vi "tcp_client.vi"() -> ()   [LabVIEW 2013]
panel:
  in  "Disconnect From Server":bool
  in  "Read From Server":bool
  in  "IP address":string
  out "Recevied Value":T1 {"Word 3" format="%x"; "Word 2" format="%x"; "Word 1" format="%x"}
  out "error out":errorcluster
  in  "Port":u16
  # "Basic client server test.  Labview is the client. Run to connect, then use the two buttons below to read\nfrom the server and/or disconnect.  The server is set up now to just send sequential numbers - this \nis a placeholder until it actually does some processing."
  # "IP Address might be 127.0.0.1 to test a server running on the same machine as Labview\nOr it could be the IP address of the TK1 board once that is up and running"
  # "Port is arbitrary - make it a number above 49152. Start the server using that same port number. It has to be unique on the machine running the server, but not unique over the whole internet."
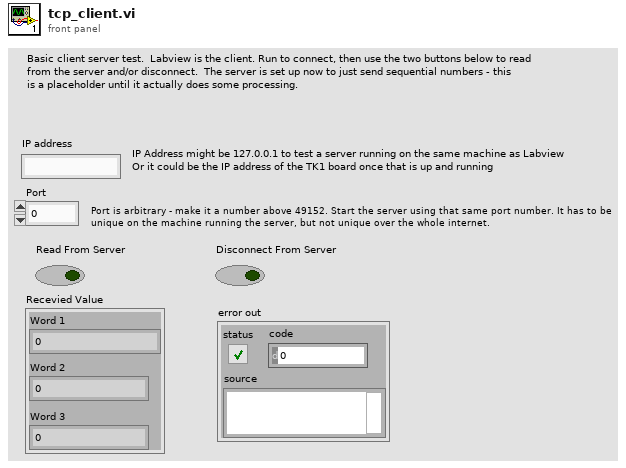
[diagram p1: front panel]
types:
  T1 = cluster{"Word 1":u32, "Word 2":u32, "Word 3":u32}
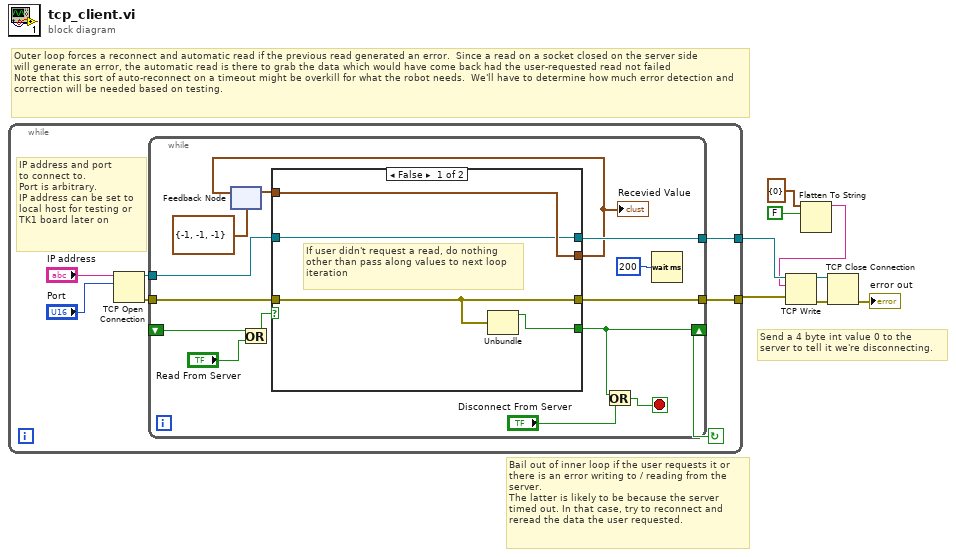
[diagram p0: block diagram]
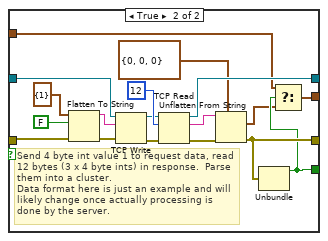
[diagram p2: hidden frame]
diagram:
  # "Send a 4 byte int value 0 to the\nserver to tell it we're disconnecting."
  # "Bail out of inner loop if the user requests it or\nthere is an error writing to / reading from the \nserver.\nThe latter is likely to be because the server\ntimed out. In that case, try to reconnect and \nreread the data the user requested."
  # "Outer loop forces a reconnect and automatic read if the previous read generated an error.  Since a read on a socket closed on the server side\nwill generate an error, the automatic read is there to grab the data which would have come back had the user-requested read not failed\nNote that this sort of auto-reconnect on a timeout might be overkill for what the robot needs.  We'll have to determine how much error detection and correction will be needed based on testing."
  n1 = while {
    tunnel: [w11] -> w3
    tunnel: [w10] -> w2
    stop <- w9 continue-if-true
    # "IP address and port\nto connect to.\nPort is arbitrary.\nIP address can be set to local host for testing or\nTK1 board later on"
    n2 = TCP Open Connection(address="IP address", remote port or service name="Port") -> (connection ID=w12:refnum<k5>, error out=w13:errorcluster)  [unwired: 3 in]
    n3 = while {
      tunnel: w13 -> [w29]
      tunnel: w12 -> [w28]
      tunnel: [w25] -> w11
      tunnel: [w26] -> w10
      shift-right: [w18] -> w9
      shift-left: _ -> [w21]
      stop <- w24 stop-if-true
      n4 = feedback #1(cluster{i32, i32, i32} {-1, -1, -1}) -> (w19:cluster{u32, u32, u32})
      n5 = Or(x=w21, y="Read From Server") -> (x .or. y?=w20:bool)
      n6 = case shown="False" w20 {
        tunnel: [w33 w36] -> w17
        tunnel: w29 -> [w31 w40]
        tunnel: w28 -> [w32 w49]
        tunnel: [w32 w46] -> w26
        tunnel: [w31 w38] -> w25
        tunnel: w19 -> [w33 w35]
        tunnel: [w30 w37] -> w18
        frame False {
          # "If user didn't request a read, do nothing\nother than pass along values to next loop\niteration"
          n7 = Unbundle(w31) -> ("status"=w30:bool)  [unwired: 2 out]
        }
        frame True {
          # "Send 4 byte int value 1 to request data, read 12 bytes (3 x 4 byte ints) in response.  Parse them into a cluster.  \nData format here is just an example and will likely change once actually processing is done by the server."
          n8 = Flatten To String(anything=cluster{u32} {1}, prepend array or string size? (T)=FALSE, error in (no error)=w40) -> (data string=w43:string, error out=w39:errorcluster)  [unwired: 1 in, 1 out]
          n9 = TCP Write(connection ID=w49, data in=w43, error in (no error)=w39) -> (connection ID out=w48:refnum<k5>, error out=w47:errorcluster)  [unwired: 1 in, 1 out]
          n10 = TCP Read(connection ID=w48, bytes to read=12, error in (no error)=w47) -> (connection ID out=w46:refnum<k5>, data out=w50:string, error out=w41:errorcluster)  [unwired: 2 in]
          n11 = Unflatten From String(type=cluster{u32, u32, u32} {0, 0, 0}, binary string=w50, error in (no error)=w41) -> (value=w34:cluster{u32, u32, u32}, error out=w38:errorcluster)  [unwired: 2 in, 1 out]
          n12 = Unbundle(w38) -> ("status"=w37:bool)  [unwired: 2 out]
          n13 = Select(t=w35, s=w37, f=w34) -> (s? t:f=w36:cluster{u32, u32, u32})
        }
      }
      "Recevied Value" <- w17
      n14 = feedback-in #1(w17) -> ()
      n15 = Or(x=w18, y="Disconnect From Server") -> (x .or. y?=w24:bool)
      n16 = Wait (ms)(milliseconds to wait=u32 200) -> ()  [unwired: 1 out]
    }
  }
  n17 = Flatten To String(anything=cluster{i32} {0}, prepend array or string size? (T)=FALSE) -> (data string=w1:string)  [unwired: 2 in, 2 out]
  n18 = TCP Write(connection ID=w2, data in=w1, error in (no error)=w3) -> (connection ID out=w5:refnum<k5>, error out=w4:errorcluster)  [unwired: 1 in, 1 out]
  n19 = TCP Close Connection(connection ID=w5, error in (no error)=w4) -> (error out=→"error out":errorcluster)  [unwired: 1 in, 1 out]
